vi "Get Setting - Main_Window_Title.vi"(8 "Error In":errorcluster) -> (0 "Error Out":errorcluster, 3 "Main_Window_Title":string)   [LabVIEW 2016, in "Error Manager.lvlib" / "Settings.lvclass"]
uses:
  Settings.lvclass
  Settings (class variable).vi
panel:
  # "Input\nInputs to the VI"
  # "Development\nControls or indicators that are useful for development or testing, but which are not outputs of the VI."
  # "Output\nOutputs of the VI"
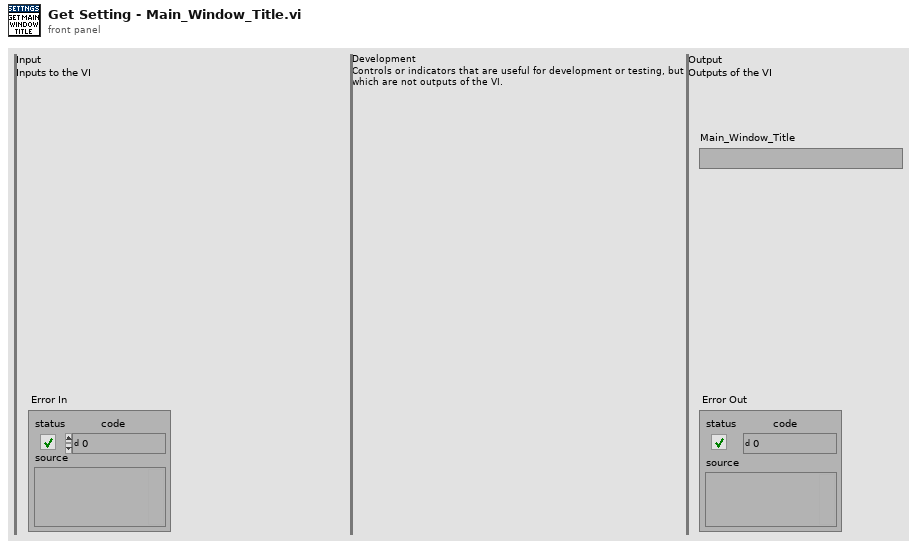
[diagram p1: front panel]
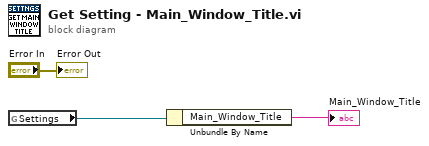
[diagram p0: block diagram]
diagram:
  n1 = global read "Settings (class variable).vi" "Settings"() -> (w1:refnum<class "Settings.lvclass">)
  n2 = Unbundle By Name(w1) -> ("Main_Window_Title"=→"Main_Window_Title":string)
  "Error Out" <- "Error In"
